vi "ProportionalResize.vi"(8 "error in (no error)":errorcluster, 11 "Refnum in":T1) -> (0 "error out":errorcluster, 2 "Size Ratio":dbl, 3 "Refnum out":T1)   [LabVIEW 2017, in "ImageAcquisitionLibrary.lvlib"]
uses:
  ImageAcquisitionLibrary.lvlib
  <vilib>/vision/Image Controls.llb/IMAQ Image.ctl
  <vilib>/vision/NI_Vision_Development_Module.lvlib
panel:
  out "Image 2":T1(plugin-control)
  out "Image":T1(plugin-control)
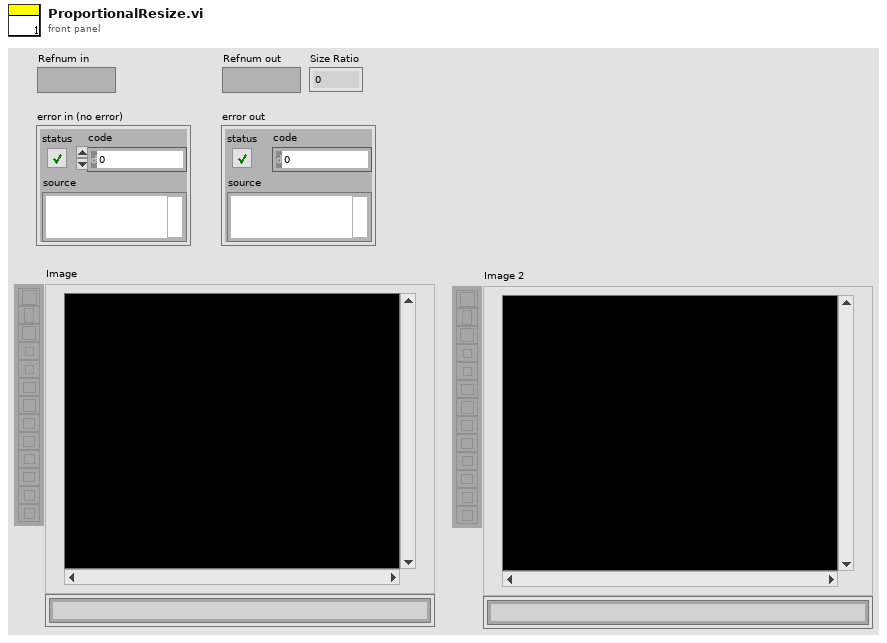
[diagram p1: front panel]
types:
  T1 = typedef "IMAQ Image.ctl" = refnum<image>
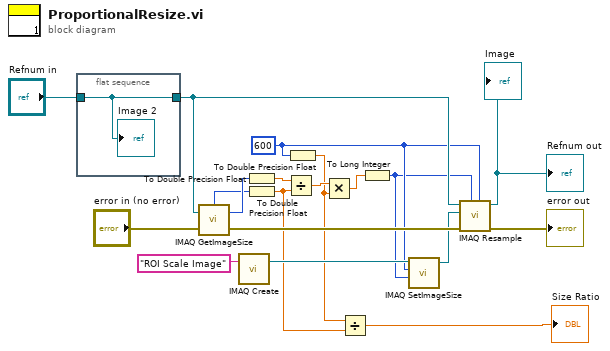
[diagram p0: block diagram]
diagram:
  w9 = 600
  n1 = flat-sequence {
    tunnel: "Refnum in" -> [w20]
    tunnel: [w20] -> w15
    frame #0 {
      "Image 2" <- w20
    }
  }
  n2 = call "IMAQ GetImageSize"("Image"=w15, "error in (no error)"="error in (no error)") -> ("Y Resolution"=w18:i32, "X Resolution"=w17:i32, "error out"=w13:errorcluster)  [unwired: 2 in]
  n3 = call "IMAQ Create"("Image Name"="ROI Scale Image") -> ("New Image"=w11:T1)  [unwired: 4 in, 1 out]
  n4 = To Double Precision Float(number=w18) -> (double precision float=w5:dbl)
  n5 = To Double Precision Float(number=w17) -> (double precision float=w3:dbl)
  n6 = Divide(x=w5, y=w3) -> (x/y=w7:dbl)
  n7 = To Double Precision Float(number=w9) -> (double precision float=w2:dbl)
  n8 = Multiply(x=w7, y=w2) -> (x*y=w6:dbl)
  n9 = Divide(x=w2, y=w3) -> (x/y=→"Size Ratio":dbl)
  n10 = To Long Integer(number=w6) -> (32bit integer=w8:i32)
  n11 = call "IMAQ SetImageSize"("Y Resolution"=w8, "X Resolution"=w9, "Image"=w11) -> ("Image Out"=w10:T1)  [unwired: 2 in, 1 out]
  n12 = call "IMAQ Resample"("X Resolution"=w9, "Y Resolution"=w8, "error in (no error)"=w13, "Image Dst"=w10, "Image Src"=w15) -> ("error out"=→"error out":errorcluster, "Image Dst Out"=→"Refnum out" →"Image":T1)  [unwired: 5 in]
